vi "turret math.vi"(9 "Current Position (native units)":dbl, 10 "Gear Ratio":dbl) -> (3 "New setpoint":dbl)   [LabVIEW 2019]
panel:
  in  "position(deg 0-360)":dbl
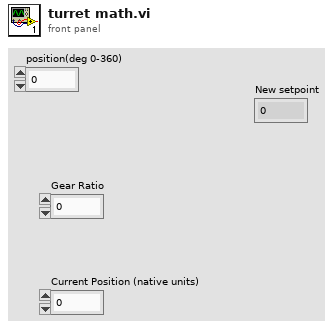
[diagram p1: front panel]
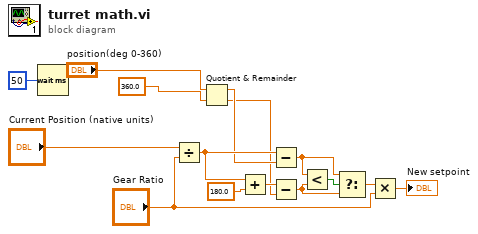
[diagram p0: block diagram]
diagram:
  n1 = Wait (ms)(milliseconds to wait=u32 50) -> ()  [unwired: 1 out]
  n2 = Divide(x="Current Position (native units)", y="Gear Ratio") -> (x/y=w10:dbl)
  n3 = Quotient & Remainder(x="position(deg 0-360)", y=360.0) -> (x-y*floor(x/y)=w2:dbl, floor(x/y)=w1:dbl)
  n4 = Add(x=w10, y=180.0) -> (x+y=w14:dbl)
  n5 = Subtract(x=w10, y=w2) -> (x-y=w12:dbl)
  n6 = Subtract(x=w14, y=w1) -> (x-y=w11:dbl)
  n7 = Less?(x=w12, y=w11) -> (x < y?=w13:bool)
  n8 = Select(t=w12, s=w13, f=w11) -> (s? t:f=w9:dbl)
  n9 = Multiply(x=w9, y="Gear Ratio") -> (x*y=→"New setpoint":dbl)
